vi "OnOff.vi"() -> ()   [LabVIEW 2020]
panel:
  out "error out":errorcluster
  in  "error in (no error)":errorcluster
  in  "VISA resource name":refnum<visa-resource-name>
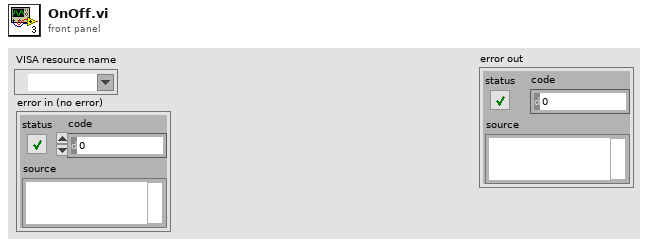
[diagram p1: front panel]
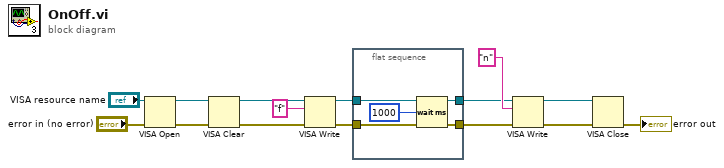
[diagram p0: block diagram]
diagram:
  n1 = VISA Open(error in (no error)="error in (no error)", VISA resource name="VISA resource name") -> (VISA resource name=w10:refnum<visa-resource-name>, error out=w15:errorcluster)  [unwired: 3 in]
  n2 = VISA Clear(VISA resource name=w10, error in (no error)=w15) -> (VISA resource name out=w9:refnum<visa-resource-name>, error out=w14:errorcluster)
  n3 = VISA Write(VISA resource name=w9, write buffer="f", error in (no error)=w14) -> (VISA resource name out=w8:refnum<visa-resource-name>, error out=w13:errorcluster)  [unwired: 1 out]
  n4 = flat-sequence {
    tunnel: w8 -> [w18]
    tunnel: [w18] -> w2
    tunnel: [w17] -> w1
    tunnel: w13 -> [w17]
    frame #0 {
      n5 = Wait (ms)(milliseconds to wait=u32 1000) -> ()  [unwired: 1 out]
    }
  }
  n6 = VISA Write(VISA resource name=w2, write buffer="n", error in (no error)=w1) -> (VISA resource name out=w6:refnum<visa-resource-name>, error out=w5:errorcluster)  [unwired: 1 out]
  n7 = VISA Close(VISA resource name=w6, error in (no error)=w5) -> (error out=→"error out":errorcluster)
